vi "DSF.Engine.Runtime.Framework.Initialize Builders.vi"(8 "error in (no error)":errorcluster, 11 "Framework Runtime in":refnum<class "DSF.Engine.Runtime.Framework.lvclass">) -> (0 "error out":errorcluster, 3 "Framework Runtime out":refnum<class "DSF.Engine.Runtime.Framework.lvclass">)   [LabVIEW 2016, in "DSF.Engine.lvlib" / "DSF.Engine.Runtime.Framework.lvclass"]
uses:
  DSF.Engine.Runtime.Framework.lvclass
  DSF.Engine.Runtime.Framework.lvclass/DSF.Engine.Runtime.Framework.ctl
  Hardware/DSF.Engine.Hardware Info.lvclass/DSF.Engine.Hardware Info.ctl
  Hardware/DSF.Engine.Hardware Info.CPU.lvclass/DSF.Engine.Hardware Info.CPU.ctl
  BuilderManager/DSF.Engine.BuilderManager.lvclass
  Hardware/DSF.Engine.Hardware Info.lvclass
  Hardware/DSF.Engine.Hardware Info.CPU.lvclass
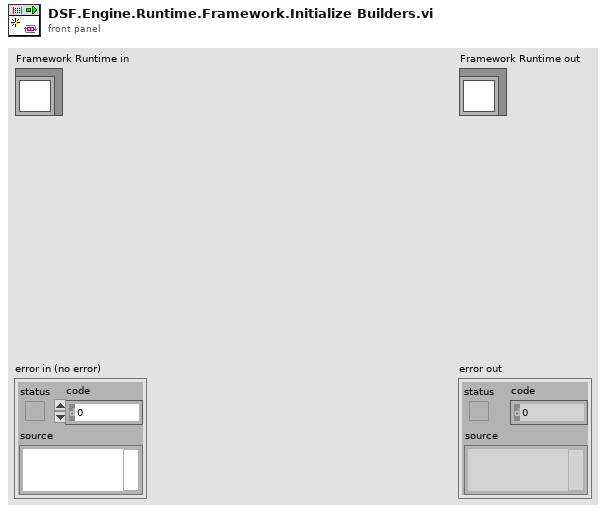
[diagram p1: front panel]
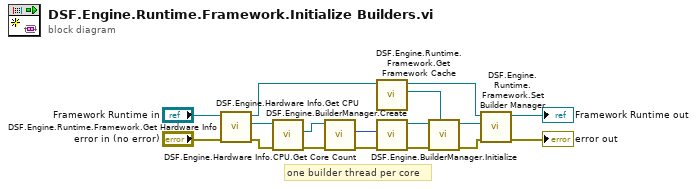
[diagram p0: block diagram]
diagram:
  # "one builder thread per core"
  n1 = call "DSF.Engine.Runtime.Framework.Get Hardware Info.vi"("error in (no error)"="error in (no error)", "Framework Runtime in"="Framework Runtime in") -> ("error out"=w10:errorcluster, "Hardware Info"=w13:refnum<class "DSF.Engine.Hardware Info.lvclass">, "Framework Runtime out"=w3:refnum<class "DSF.Engine.Runtime.Framework.lvclass">)  [unwired: 7 in]
  n2 = call "DSF.Engine.Hardware Info.Get CPU.vi"("error in (no error)"=w10, "Hardware Info in"=w13) -> ("error out"=w11:errorcluster, "CPU Info"=w12:refnum<class "DSF.Engine.Hardware Info.CPU.lvclass">)  [unwired: 7 in, 1 out]
  n3 = call "DSF.Engine.Hardware Info.CPU.Get Core Count.vi"("error in (no error)"=w11, "CPU Info in"=w12) -> ("error out"=w8:errorcluster, "Core Count"=w9:i32)  [unwired: 7 in, 1 out]
  n4 = call "DSF.Engine.Runtime.Framework.Get Framework Cache.vi"("Framework Runtime in"=w3) -> ("Framework Cache"=w1:refnum<class "DSF.Engine.Memory.Cache.Framework.lvclass">, "Framework Runtime out"=w2:refnum<class "DSF.Engine.Runtime.Framework.lvclass">)  [unwired: 8 in, 1 out]
  n5 = call "DSF.Engine.BuilderManager.Create.vi"("error in (no error)"=w8, "number of builders"=w9) -> ("error out"=w6:errorcluster, "Builder Manager"=w7:refnum<class "DSF.Engine.BuilderManager.lvclass">)  [unwired: 8 in]
  n6 = call "DSF.Engine.BuilderManager.Initialize.vi"("Framework Cache"=w1, "error in (no error)"=w6, "Builder Manager in"=w7) -> ("error out"=w5:errorcluster, "Builder Manager out"=w4:refnum<class "DSF.Engine.BuilderManager.lvclass">)  [unwired: 7 in]
  n7 = call "DSF.Engine.Runtime.Framework.Set Builder Manager.vi"("error in (no error)"=w5, "Builder Manager"=w4, "Framework Runtime in"=w2) -> ("error out"=→"error out":errorcluster, "Framework Runtime out"=→"Framework Runtime out":refnum<class "DSF.Engine.Runtime.Framework.lvclass">)  [unwired: 7 in]
